vi "_Obtain CSM Data Queue.vi"(8 "error in (no error)":errorcluster, 9 "create if not found? (T)":bool=TRUE, 11 "Name":string) -> (0 "error out":errorcluster, 1 "created new?":bool, 3 "Priority Queue":refnum<class "Priority Queue.lvclass">)   [LabVIEW 2020, in "Communicable State Machine.lvlib"]
uses:
  Communicable State Machine.lvlib
  Priority Queue.lvclass
  Priority Queue.lvclass/Priority Queue.ctl
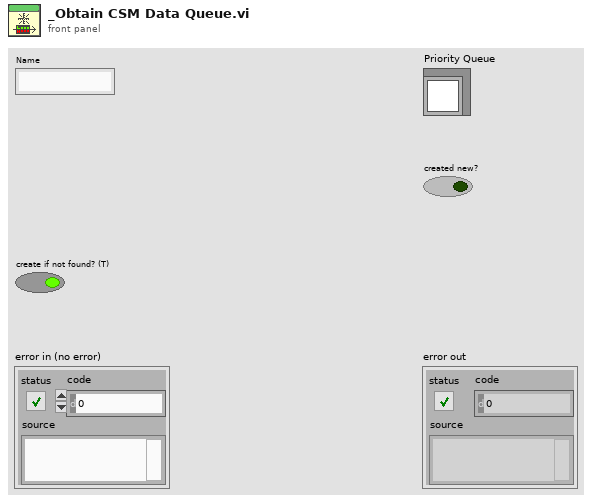
[diagram p1: front panel]
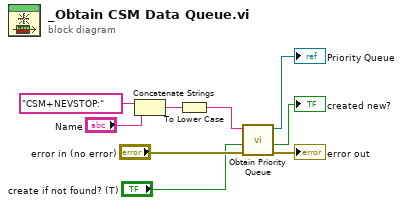
[diagram p0: block diagram]
diagram:
  n1 = Concatenate Strings("CSM+NEVSTOP:" ("string"), "Name") -> (w8:string)
  n2 = To Lower Case(string=w8) -> (all lower case string=w1:string)
  n3 = call "Obtain Priority Queue.vi"("error in (no error)"="error in (no error)", "create if not found? (T)"="create if not found? (T)", "name"=w1) -> ("error out"=→"error out":errorcluster, "created new?"=→"created new?":bool, "Priority Queue"=→"Priority Queue":refnum<class "Priority Queue.lvclass">)  [unwired: 6 in]
